vi "Strain Gauge.vi"(11 "Queue ref":T1) -> ()   [LabVIEW 2022 SP3]
uses:
  Controls/All Queue.ctl
  Controls/DAQ case.ctl
  Controls/UI Data.ctl
  Controls/All Loop Status.ctl
  <vilib>/DAQmx/read.llb/DAQmx Read (Analog 1D Wfm NChan NSamp).vi
  Create Task/Strain Create Task.vi
  <vilib>/DAQmx/configure/timing.llb/DAQmx Timing (Sample Clock).vi
  Sub VI's/Global 1.vi
  <vilib>/DAQmx/miscellaneous.llb/DAQmx Fill In Error Info.vi
panel:
  out "error IO":errorcluster
  # "TC channel list"
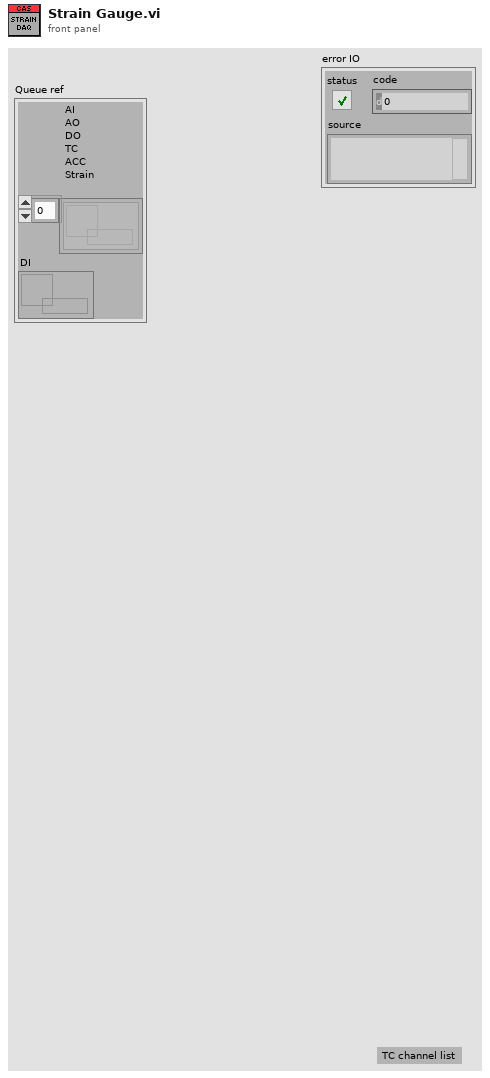
[diagram p1: front panel]
types:
  T1 = typedef "All Queue.ctl" = cluster{"AI\nAO\nDO\nTC\nACC\nStrain":refnum<queue>[], "DI":refnum<queue>}
  T2 = cluster{"in progress?":bool, "Queue ref":T1, "Start DAQ":refnum<notifier>, "UI Data":refnum<notifier>, "task out":refnum<k21>, "SG Ref":refnum<queue>, "SPC":i32}
  T3 = typedef "DAQ case.ctl" = enum16{"Initailise", "Create Task", "Polevent", "Acquire", "Stop DAQ", "Error", "Exit"}
  T4 = typedef "All Loop Status.ctl" = enum16{"AI", "AO", "DI", "DO", "TC", "Strain", "ACC", "RT", "Log"}
  T5 = enum16{"Init", "Read 'All'", "Read 'n'", "Read '1'", "Write '1'", "Write 'n'", "Write 'All'"}
  T6 = typedef "All Notifer.ctl" = cluster{"UI Data":refnum<notifier>, "Start DAQ":refnum<notifier>, "Start Log":refnum<notifier>}
  T7 = cluster{"Analog input":bool, "Analog Output":bool, "Digital input":bool, "Digital output":bool, "Thermocouple":bool, "Strain Gauge":bool, "Accelerometer":bool}
  T8 = typedef "Config.ctl" = cluster{"AO config":cluster{"Channel_Name":string, "Channel_Number":string, "Default_Value":dbl, "Units":string}[], "AI config":cluster{"Channel_Name":string, "Channel_Number":string, "Pre_Scale_min":dbl, "Pre_Scale_max":dbl, "Sensor_min":dbl, "Sensor_max":dbl, "Units":string}[], "DI config":cluster{"Channel_Name":string, "Channel_Number":string, "Default_Value":bool, "DI invert?":bool}[], "DO config":cluster{"Channel_Name":string, "Channel_Number":string, "Default_Value":bool, "DO invert?":bool}[], "TC config":cluster{"Channel_Name":string, "Channel_Number":string, "Pre_Scale_min":dbl, "Pre_Scale_max":dbl, "units":i32, " type":i32}[], "ACC config":cluster{"Channel_Name":string, "Channel_Number":string, "Pre_Scale_min":dbl, "Pre_Scale_max":dbl, "Terminal configuration":i32, "Sensitivity":dbl, "Sensitivity units":i32}[], "SG config":cluster{"Channel_Name":string, "Channel_Number":string, "Pre_Scale_min":dbl, "Pre_Scale_max":dbl}[], "Strain Gauge Settings":cluster{"poisson ratio":dbl, "nominal gage resistance":dbl, "gage factor":dbl}, "bridge information":cluster{"strain configuration":i32, "lead wire resistance":dbl, "initial bridge voltage":dbl, "voltage excitation source":i32, "voltage excitation value":dbl}, "Sample Rate":cluster{"AI Sample Rate":dbl, "AO Sample Rate":dbl, "DI Sample Rate":dbl, "TC Sample Rate":dbl, "DO Sample Rate":dbl, "SG Sample Rate":dbl, "ACC Sample Rate":dbl}}
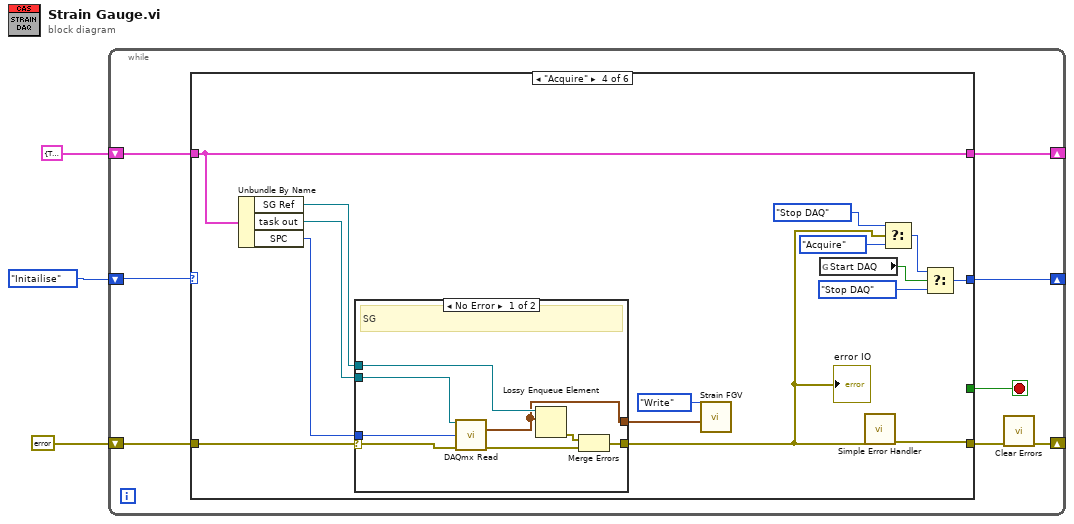
[diagram p0: block diagram]
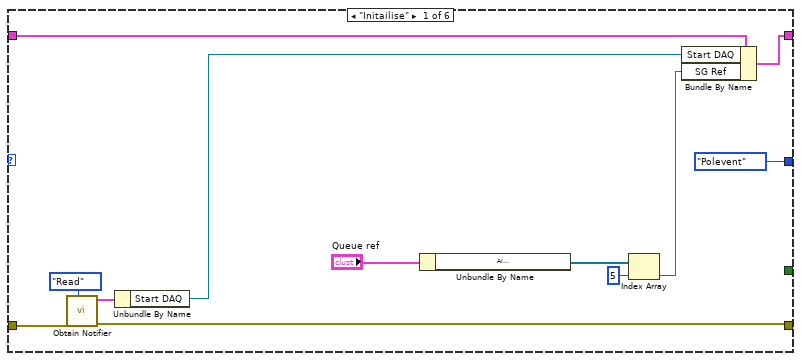
[diagram p2: hidden frame]
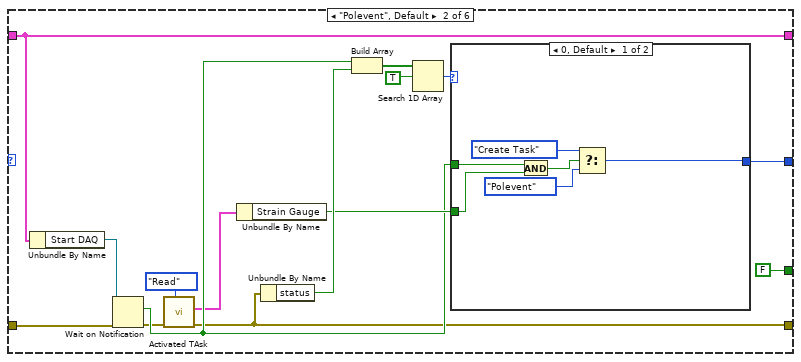
[diagram p3: hidden frame]
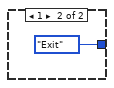
[diagram p4: hidden frame]
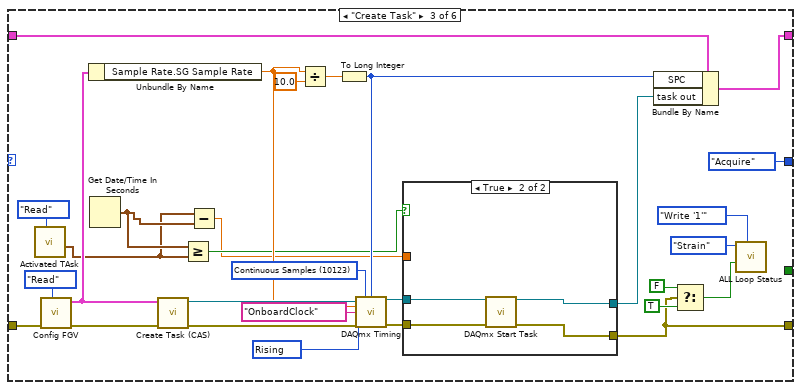
[diagram p5: hidden frame]
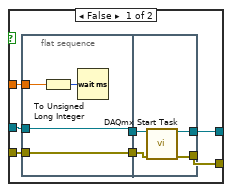
[diagram p6: hidden frame]
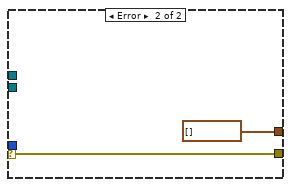
[diagram p7: hidden frame]
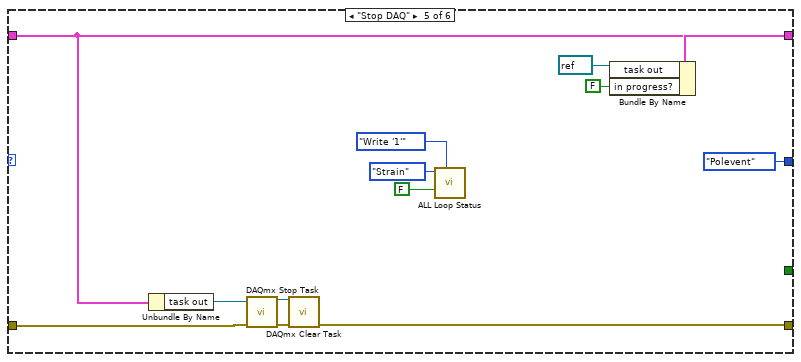
[diagram p8: hidden frame]
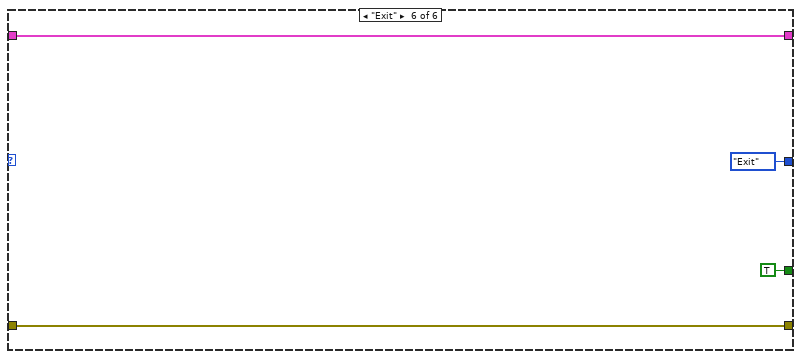
[diagram p9: hidden frame]
diagram:
  n1 = while {
    shift-right: [w4] -> _
    shift-left: errorcluster {"status"=FALSE, "code"=0, "source"=""} ("error out") -> [w10]
    shift-right: [w8] -> _
    shift-left: T2 {"in progress?"=TRUE, "Queue ref"={"AI\nAO\nDO\nTC\nACC\nStrain"=[], "DI"=refnum}, "Start DAQ"=refnum, "UI Data"=refnum, "task out"="", "SG Ref"=refnum, "SPC"=0} -> [w9]
    shift-right: [w7] -> _
    shift-left: DAQ_case."Initailise" -> [w6]
    stop <- w11 stop-if-true
    n2 = case shown="\"Acquire\"" w6 {
      tunnel: [_ FALSE _ _ _ TRUE] -> w11
      tunnel: w10 -> [w22 w27 w72 w102 w124 w136]
      tunnel: [w21 w25 w53 w96 w125 w136] -> w5
      tunnel: w9 -> [w19 w36 w74 w103 w129 w135]
      tunnel: [w17 w36 w73 w103 w130 w135] -> w8
      tunnel: [DAQ_case."Polevent" w37 DAQ_case."Acquire" w104 DAQ_case."Polevent" DAQ_case."Exit"] -> w7
      frame "Initailise" {
        n3 = call "Obtain Notifier.vi"("Case"=enum16{"Obtain", "Read"}."Read", "error in (no error)"=w22) -> ("error out"=w21:errorcluster, "notifiers out"=w20:T6)  [unwired: 8 in]
        n4 = Unbundle By Name(w20) -> ("Start DAQ"=w18:refnum<notifier>)
        n5 = Unbundle By Name("Queue ref") -> ("AI\nAO\nDO\nTC\nACC\nStrain"=w14:refnum<queue>[])
        n6 = Index Array(array=w14, index=5) -> (element=w13:refnum<queue>)
        n7 = Bundle By Name(cluster=w19, "Start DAQ"=w18, "SG Ref"=w13) -> (w17:T2)
      }
      frame "Polevent", Default {
        n8 = Unbundle By Name(w36) -> ("Start DAQ"=w35:refnum<notifier>)
        n9 = Wait on Notification(notifier=w35, error in (no error)=w27) -> (notification=w28:bool, error out=w26:errorcluster)  [unwired: 2 in, 2 out]
        n10 = call "Activated TAsk.vi"("Enum"=enum16{"Read", "Write"}."Read", "error in (no error)"=w26) -> ("error out"=w25:errorcluster, "Activate Task 2"=w24:T7)  [unwired: 7 in, 1 out]
        n11 = Unbundle By Name(w24) -> ("Strain Gauge"=w29:bool)
        n12 = Unbundle By Name(w25) -> ("status"=w34:bool)
        n13 = Build Array(w28, w34) -> (w33:bool[])
        n14 = Search 1D Array(1D array=w33, element=TRUE) -> (index of element=w31:i32)  [unwired: 1 in]
        n15 = case shown="0, Default" w31 {
          tunnel: [w43 DAQ_case."Exit"] -> w37
          tunnel: w29 -> [w40 _]
          tunnel: w28 -> [w39 _]
          frame 0, Default {
            n16 = And(x=w39, y=w40) -> (x .and. y?=w41:bool)
            n17 = Select(t=DAQ_case."Create Task", s=w41, f=DAQ_case."Polevent") -> (s? t:f=w43:T3)
          }
          frame 1 {
          }
        }
      }
      frame "Create Task" {
        w46 = 10280 items=["Rising"=10280, "Falling"=10171] ("active edge")
        w66 = 10123 items=["Finite Samples"=10178, "Continuous Samples"=10123, "Hardware Timed Single Point"=12522] ("sample mode")
        n18 = call "Activated TAsk.vi"("Enum"=enum16{"Read", "Write"}."Read") -> ("Start Time"=w48:timestamp)  [unwired: 8 in, 2 out]
        n19 = call "Config FGV.vi"("Enum"=enum16{"Read", "Write"}."Read", "error in (no error)"=w72) -> ("error out"=w69:errorcluster, "Data"=w60:T8)  [unwired: 8 in]
        n20 = Unbundle By Name(w60) -> ("Sample Rate.SG Sample Rate"=w59:dbl)
        n21 = Get Date/Time In Seconds() -> (seconds since 1Jan1904=w49:timestamp)
        n22 = call-poly "Create Task (CAS).vi"("error in"=w69, "Data"=w60) -> ("error out"=w67:errorcluster, "task out"=w68:refnum<k21>)  [unwired: 7 in, 1 out]
        n23 = Greater Or Equal?(x=w49, y=w48) -> (x >= y?=w51:bool)
        n24 = Subtract(x=w48, y=w49) -> (x-y=w50:dbl)
        n25 = Divide(x=w59, y=10.0) -> (x/y=w57:dbl)
        n26 = To Long Integer(number=w57) -> (32bit integer=w56:i32)
        n27 = call-poly <vilib>:"DAQmx Timing.vi"("task/channels in"=w68, "sample mode"=w66, "samples per channel"=w56, "rate"=w59, "source"=tag "OnboardClock", "active edge"=w46, "error in"=w67) -> ("task out"=w55:refnum<k21>, "error out"=w54:errorcluster)  [unwired: 7 in]
        n28 = case shown="True" w51 {
          tunnel: [w82 w94] -> w53
          tunnel: [w81 w93] -> w52
          tunnel: w55 -> [w80 w92]
          tunnel: w54 -> [w79 w91]
          tunnel: w50 -> [w76 _]
          frame False {
            n29 = flat-sequence {
              tunnel: w80 -> [w84]
              tunnel: w79 -> [w85]
              tunnel: [w85] -> w78
              tunnel: [w84] -> w77
              tunnel: w76 -> [w83]
              tunnel: [w90] -> w82
              tunnel: [w89] -> w81
              tunnel: w78 -> [w88]
              tunnel: w77 -> [w87]
              frame #0 {
                n30 = To Unsigned Long Integer(number=w83) -> (unsigned 32bit integer=w86:u32)
                n31 = Wait (ms)(milliseconds to wait=w86) -> ()  [unwired: 1 out]
              }
              frame #1 {
                n32 = call <vilib>:"DAQmx Start Task.vi"("task/channels in"=w87, "error in"=w88) -> ("task out"=w89:refnum<k21>, "error out"=w90:errorcluster)  [unwired: 12 in]
              }
            }
          }
          frame True {
            n33 = call <vilib>:"DAQmx Start Task.vi"("task/channels in"=w92, "error in"=w91) -> ("task out"=w93:refnum<k21>, "error out"=w94:errorcluster)  [unwired: 12 in]
          }
        }
        n34 = Bundle By Name(cluster=w74, "SPC"=w56, "task out"=w52) -> (w73:T2)
        n35 = Select(t=FALSE, s=w53, f=TRUE) -> (s? t:f=w63:bool)
        n36 = call "ALL Loop Status.vi"("Option"=T5."Write '1'", "Status"=w63, "Loop"=All_Loop_Status."Strain") -> ()  [unwired: 6 in, 3 out]
      }
      frame "Acquire" {
        n37 = Unbundle By Name(w103) -> ("SG Ref"=w101:refnum<queue>, "task out"=w100:refnum<k21>, "SPC"=w95:i32)
        n38 = case shown="No Error" w102 {
          selector: w102 -> [w114 w119]
          tunnel: w100 -> [w113 _]
          tunnel: [w116 w119] -> w97
          tunnel: w101 -> [w115 _]
          tunnel: [w112 waveform(dbl)[] [] ("data")] -> w98
          tunnel: w95 -> [w110 _]
          frame No Error {
            # "SG"
            n39 = call-poly <vilib>:"DAQmx Read.vi"("task/channels in"=w113, "number of samples per channel"=w110, "error in"=w114) -> ("data"=w112:waveform(dbl)[], "error out"=w117:errorcluster)  [unwired: 10 in, 1 out]
            n40 = Lossy Enqueue Element(queue=w115, element=w112) -> (error out=w111:errorcluster)  [unwired: 1 in, 3 out]
            n41 = Merge Errors(w111, w117) -> (w116:errorcluster)
          }
          frame Error {
          }
        }
        "error IO" <- w97
        n42 = call "Strain FGV.vi"("AI data"=w98, "Enum"=enum16{"Read", "Write"}."Write") -> ()  [unwired: 9 in, 1 out]
        n43 = global read "Global 1.vi" "Start DAQ"() -> (w107:bool)
        n44 = call <vilib>:"Simple Error Handler.vi"("error in (no error)"=w97) -> ("error out"=w96:errorcluster)  [unwired: 4 in, 4 out]
        n45 = Select(t=DAQ_case."Stop DAQ", s=w97, f=DAQ_case."Acquire") -> (s? t:f=w106:T3)
        n46 = Select(t=w106, s=w107, f=DAQ_case."Stop DAQ") -> (s? t:f=w104:T3)
      }
      frame "Stop DAQ" {
        n47 = Unbundle By Name(w129) -> ("task out"=w123:refnum<k21>)
        n48 = call <vilib>:"DAQmx Stop Task.vi"("task/channels in"=w123, "error in"=w124) -> ("task out"=w122:refnum<k21>, "error out"=w126:errorcluster)  [unwired: 12 in]
        n49 = call <vilib>:"DAQmx Clear Task.vi"("task in"=w122, "error in"=w126) -> ("error out"=w125:errorcluster)  [unwired: 13 in]
        n50 = call "ALL Loop Status.vi"("Option"=T5."Write '1'", "Status"=FALSE, "Loop"=All_Loop_Status."Strain") -> ()  [unwired: 6 in, 3 out]
        n51 = Bundle By Name(cluster=w129, "task out"=refnum<k21> refnum, "in progress?"=FALSE) -> (w130:T2)
      }
      frame "Exit" {
      }
    }
    n52 = call <vilib>:"Clear Errors.vi"("error in (no error)"=w5) -> ("error out"=w4:errorcluster)  [unwired: 5 in, 1 out]
  }
